vi "WSVCAP SHL Host LL Manage FPGA Top Level Controls Instance Manager.vi"(4 "I/O Choice (read)":T1, 6 "FPGA":T4, 8 "error in (no error)":errorcluster, 11 "Top Level Controls In":T2) -> (0 "error out":errorcluster, 3 "Top Level Controls Out":T2)   [LabVIEW 2017]
uses:
  Type Defs/Top Level Controls Core Cluster.ctl
  Type Defs/WSVCAP SHL FPGA Ref.ctl
  Type Defs/WSVCAP SHL FPGA Enum.ctl
  user.lib/Utilities/Type Defs/MISC IO Choice Enum.ctl
panel:
  out "Top Level Controls":T2[](array[typedef])
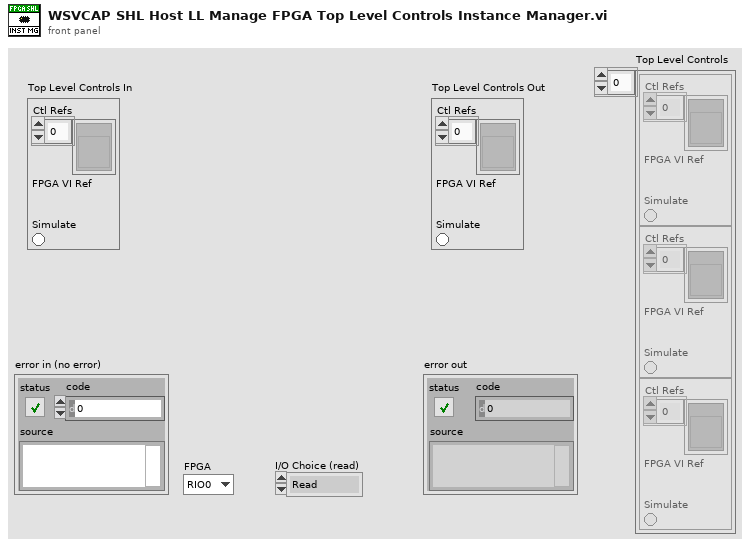
[diagram p1: front panel]
types:
  T1 = typedef "MISC IO Choice Enum.ctl" = enum16{"Read", "Write"}
  T2 = typedef "Top Level Controls Core Cluster.ctl" = cluster{"Ctl Refs":refnum<vi>[], "FPGA VI Ref":T3, "Simulate":bool}
  T3 = typedef "WSVCAP SHL FPGA Ref.ctl" = refnum<k20>
  T4 = typedef "WSVCAP SHL FPGA Enum.ctl" = enum16{"RIO0", "RIO1"}
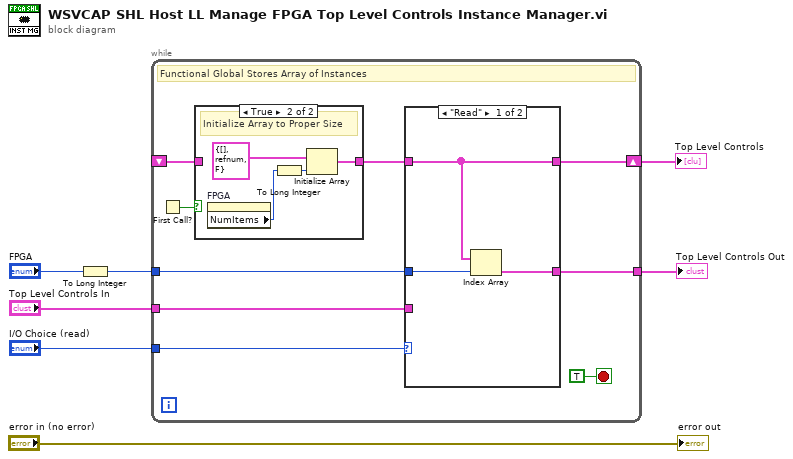
[diagram p0: block diagram]
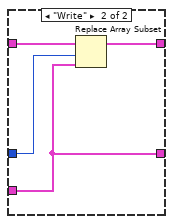
[diagram p2: hidden frame]
diagram:
  n1 = To Long Integer(number="FPGA") -> (32bit integer=w3:i32)
  n2 = while {
    shift-right: [w11] -> w5
    shift-left: _ -> [w13]
    tunnel: "I/O Choice (read)" -> [w14]
    tunnel: "Top Level Controls In" -> [w10]
    tunnel: w3 -> [w9]
    tunnel: [w8] -> w2
    stop <- TRUE ("stop") stop-if-true
    # "Functional Global Stores Array of Instances"
    n3 = First Call?() -> (First Call?: T/F=w16:bool)
    n4 = case shown="True" w16 {
      tunnel: w13 -> [w24 _]
      tunnel: [w24 w25] -> w12
      frame False {
        # "Use Stored Instances"
      }
      frame True {
        # "Initialize Array to Proper Size"
        n5 = property on="FPGA" class="Enum (strict)"() -> ("NumItems"=w27:u32)  [unwired: 2 in, 2 out]
        n6 = To Long Integer(number=w27) -> (32bit integer=w26:i32)
        n7 = Initialize Array(T2 {"Ctl Refs"=[], "FPGA VI Ref"=refnum, "Simulate"=FALSE} ("Top Level Controls In"), w26) -> (w25:T2[])
      }
    }
    n8 = case shown="\"Read\"" w14 {
      tunnel: [w17 w22] -> w11
      tunnel: w12 -> [w17 w23]
      tunnel: w10 -> [_ w20]
      tunnel: w9 -> [w19 w21]
      tunnel: [w18 w20] -> w8
      frame "Read" {
        n9 = Index Array(array=w17, index=w19) -> (element=w18:T2)
      }
      frame "Write" {
        n10 = Replace Array Subset(array=w23, new element=w20, index=w21) -> (w22:T2[])
      }
    }
  }
  "Top Level Controls" <- w5
  "Top Level Controls Out" <- w2
  "error out" <- "error in (no error)"
